vi "AddPMUModule.vi"(8 "Error In":errorcluster[](array[cluster]), 11 "Bus in":refnum<class "Bus.lvclass">) -> (0 "Error Out":errorcluster[](array[cluster]), 2 "clBroadcastEvents":T1, 3 "Bus out":refnum<class "Bus.lvclass">)   [LabVIEW 2014]
uses:
  <userlib>/NIST/NistModuleAdminLib/NistModuleAdmin/NistModuleAdmin.lvclass
  <userlib>/NIST/NISTErrorLib/NISTErrorLib.lvlib
  PmuImpairment/PmuImpairModule/Main.vi
  PmuImpairment/PmuImpairModule/PmuImpairModule.lvlib
  Bus.lvclass
  PmuImpairment/PmuImpairModule/Protected/clEventType.ctl
  PmuImpairment/PmuImpairModule/Protected/Broadcasts/clBroadcastEvents.ctl
panel:
  # "If you want to add other Broadcast Events, open this typedef, copy an existing event and rename it to your event name.\n\nNext create an \"arg\" typedef for the  data and put it into PublicAPI/Arguments/Broadcasts\n\nAfter that, you will need to create a new roadcast vi in Protected/Broadcast.  Look at DidInit.vi or the reportError.vi as examples."
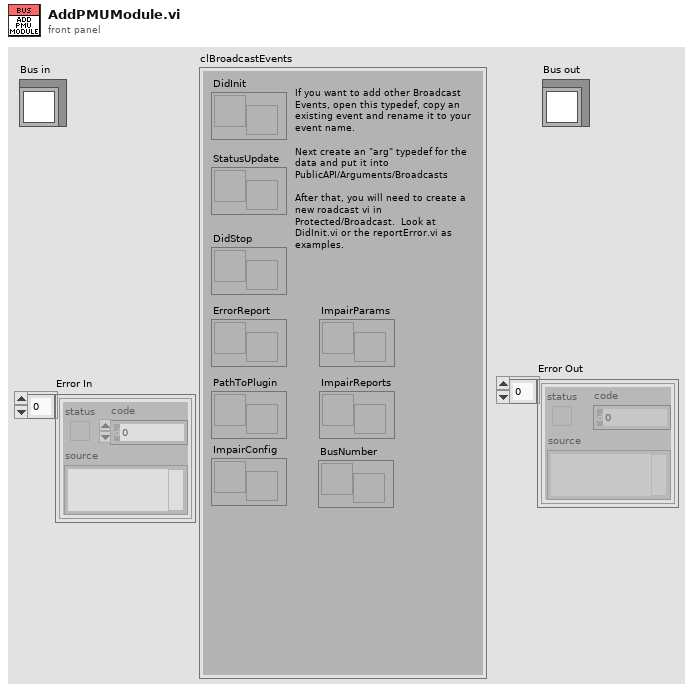
[diagram p1: front panel]
types:
  T1 = typedef "PmuImpairModule.lvlib/clBroadcastEvents.ctl" = cluster{"DidInit":refnum<user-event>, "StatusUpdate":refnum<user-event>, "ErrorReport":refnum<user-event>, "DidStop":refnum<user-event>, "ImpairConfig":refnum<user-event>, "ImpairParams":refnum<user-event>, "ImpairReports":refnum<user-event>, "PathToPlugin":refnum<user-event>, "BusNumber":refnum<user-event>}
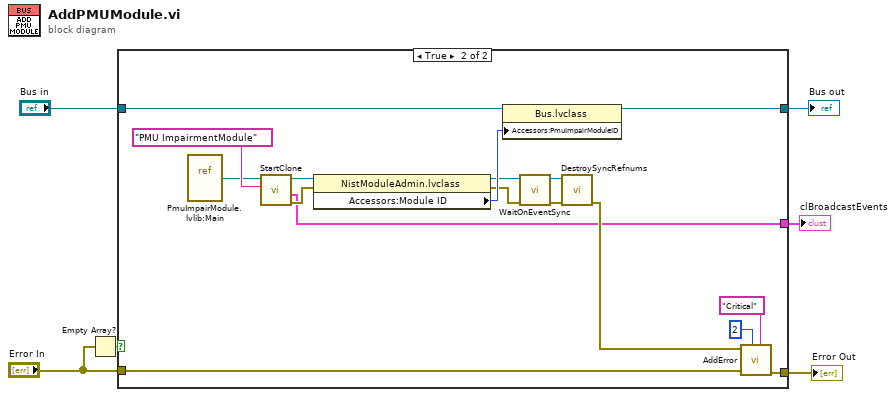
[diagram p0: block diagram]
diagram:
  n1 = Empty Array?(array="Error In") -> (empty?=w3:bool)
  n2 = case shown="True" w3 {
    tunnel: [w7 w18] -> w4
    tunnel: [w8 w24] -> w5
    tunnel: "Bus in" -> [w8 w25]
    tunnel: "Error In" -> [w7 w17]
    tunnel: [_ w9] -> w1
    frame False {
    }
    frame True {
      n3 = vi-ref "PmuImpairModule.lvlib:Main.vi"() -> (w13:refnum<vi>)
      n4 = call "StartClone.vi"("ModuleName"="PMU ImpairmentModule", "VI Refnum"=w13) -> ("error out"=w11:errorcluster, "clBroadcastEvents"=w9:T1, "ModuleAdmin"=w12:refnum<class "NistModuleAdmin.lvclass">)  [unwired: 7 in]
      n5 = property class="NistModuleAdmin.lvclass"(reference=w12, error in=w11) -> (reference out=w21:refnum<class "NistModuleAdmin.lvclass">, error out=w22:errorcluster, "Accessors:Module ID"=w23:i32)
      n6 = property class="Bus.lvclass"(reference=w25, "Accessors:PmuImpairModuleID"=w23) -> (reference out=w24:refnum<class "Bus.lvclass">)  [unwired: 1 in, 1 out]
      n7 = call <userlib>:"WaitOnEventSync.vi"("error in (no error)"=w22, "ModuleAdmin"=w21) -> ("error out"=w20:errorcluster, "ModuleAdmin"=w19:refnum<class "NistModuleAdmin.lvclass">)  [unwired: 8 in]
      n8 = call <userlib>:"DestroySyncRefnums.vi"("error in (no error)"=w20, "ModuleAdmin"=w19) -> ("error out"=w10:errorcluster)  [unwired: 9 in]
      n9 = call <userlib>:"AddError.vi"("Severity"="Critical", "Priority"=u8 2, "ErrorArray"=w17, "error in (no error)"=w10) -> ("ErrorArray"=w18:errorcluster[])  [unwired: 6 in, 1 out]
    }
  }
  "Bus out" <- w5
  "Error Out" <- w4
  "clBroadcastEvents" <- w1
